vi "Paro_for.vi"() -> ()   [LabVIEW 2016]
panel:
  in  "Stop Button":bool
  out "Numeric Control":i32
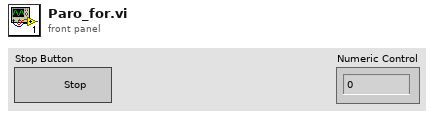
[diagram p1: front panel]
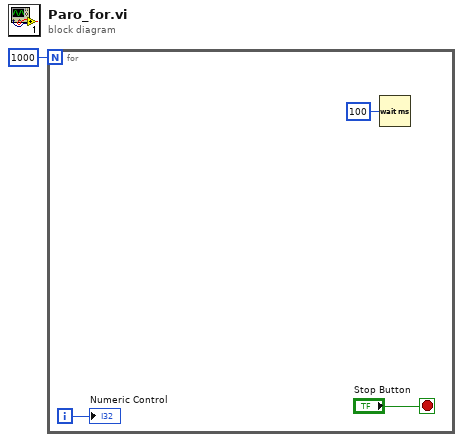
[diagram p0: block diagram]
diagram:
  n1 = for {
    N: 1000 -> [_]
    i -> [w3]
    stop <- "Stop Button" stop-if-true
    n2 = Wait (ms)(milliseconds to wait=u32 100) -> ()  [unwired: 1 out]
    "Numeric Control" <- w3
  }
